vi "Enter Key.vi"() -> (1 "Canceled?":bool, 3 "Product Key Out":string)   [LabVIEW 2012]
panel:
  in  "Cancel Button":bool
  in  "OK Button":bool
  in  "Product Key":string
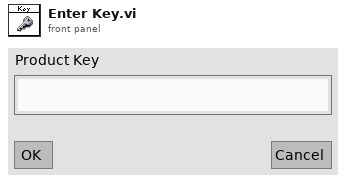
[diagram p1: front panel]
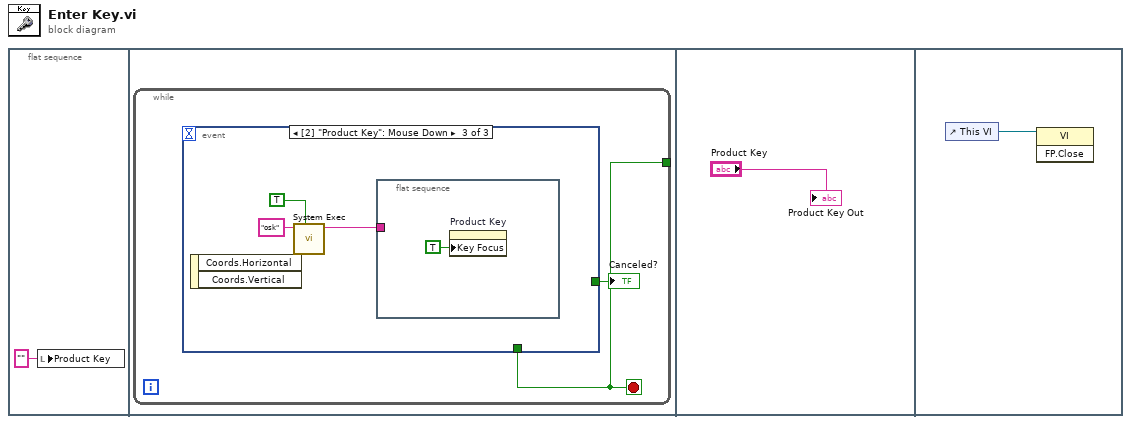
[diagram p0: block diagram]
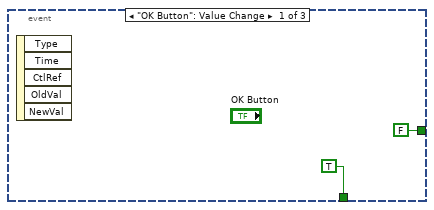
[diagram p2: hidden frame]
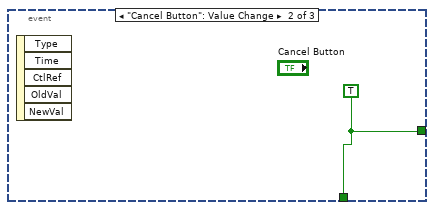
[diagram p3: hidden frame]
diagram:
  n1 = flat-sequence {
    frame #0 {
      n2 = local write "Product Key"("" ("Product Key")) -> ()
    }
    frame #1 {
      n3 = while {
        tunnel: [w3] -> _
        stop <- w3 stop-if-true
        n4 = event shown="[2] \"Product Key\": Mouse Down" {
          selector: _ -> [_ _ _]
          dyn-events: _ -> [_ _ _]
          timeout: _ -> [_ _ _]
          tunnel: [TRUE w6 _] -> w3
          tunnel: [FALSE w6 _] -> w2
          event "OK Button": Value Change {
            n5 = event-data() -> ()  [unwired: 1 in, 5 out]
          }
          event "Cancel Button": Value Change {
            w6 = TRUE
            n6 = event-data() -> ()  [unwired: 1 in, 5 out]
          }
          event "Product Key": Mouse Down {
            n7 = event-data() -> ()  [unwired: 1 in, 2 out]
            n8 = call <vilib>:"System Exec.vi"("wait until completion? (T)"=TRUE, "command line"="osk") -> ("standard output"=w7:string)  [unwired: 6 in, 3 out]
            n9 = flat-sequence {
              tunnel: w7 -> [_]
              frame #0 {
                n10 = property on="Product Key" class="Str"("Key Focus"=TRUE) -> ()  [unwired: 2 in, 2 out]
              }
            }
          }
        }
        "Canceled?" <- w2
      }
    }
    frame #2 {
      "Product Key Out" <- "Product Key"
    }
    frame #3 {
      n11 = control-ref of="This VI"() -> (w12:refnum<vi>)
      n12 = invoke class="VI" method="FP.Close"(reference=w12) -> ()  [unwired: 2 in, 3 out]
    }
  }
